vi "Pre Launch Init.vi"(11 "Test Node Charm View in":refnum<class "Test Node Charm View.lvclass">) -> (0 "error out":errorcluster, 3 "Test Node Charm View out":refnum<class "Test Node Charm View.lvclass">)   [LabVIEW 2013, in "Test Node Charm View.lvlib" / "Test Node Charm View.lvclass"]
doc: "(<B>Filename</B>: Actor Framework.lvlib:Actor.lvclass:Pre Launch Init.vi)\n\nDefines behavior that occurs after the Launch Actor method is invoked but before the actor's Actor Core method begins running.\n\nThe Pre Launch Init method is guaranteed to finish before the Launch Actor method returns to its caller and before the actor itself receives any messages. Any references that the Pre Launch Init method obtains are guaranteed to have the same lifetime as the actor itself. Any errors that the Pre Launch Init method returns will abort the launch.\n\nBy default, this method does nothing. A descendant class may override it to define behavior."
uses:
  Test Node Charm View.lvclass
  <vilib>/ActorFrameworkMVC/View Actor/View Actor.lvclass
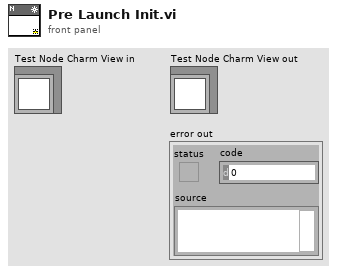
[diagram p1: front panel]
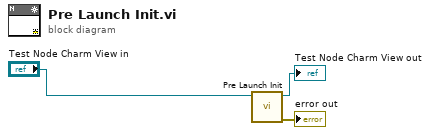
[diagram p0: block diagram]
diagram:
  n1 = call-parent "Pre Launch Init.vi"("Actor in"="Test Node Charm View in") -> ("error out"=→"error out":errorcluster, "Actor out"=→"Test Node Charm View out":refnum<class "Test Node Charm View.lvclass">)  [unwired: 9 in]
